vi "Encode Remaining Length.vi"(11 "Remaining Length (bytes)":u32) -> (2 "Valid length":bool, 3 "Encoded Remaining Length":u8[](array[numeric]) format="%02x")   [LabVIEW 2013, in "ControlPacket.lvclass"]
uses:
  ControlPacket.lvclass
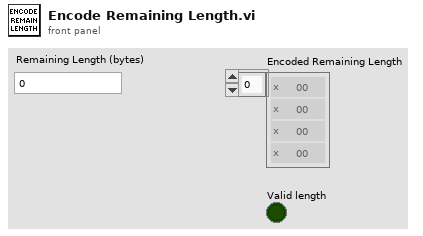
[diagram p1: front panel]
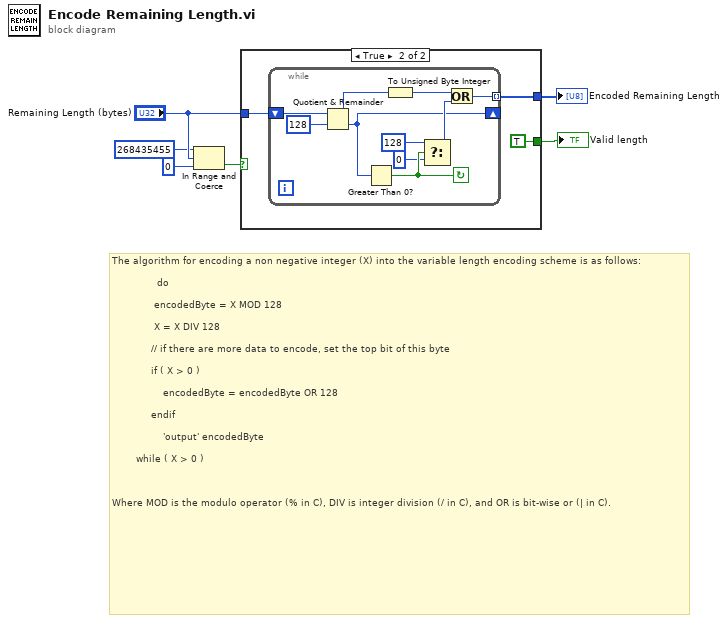
[diagram p0: block diagram]
diagram:
  # "The algorithm for encoding a non negative integer (X) into the variable length encoding scheme is as follows:\n\n               do\n\n              encodedByte = X MOD 128\n\n              X = X DIV 128\n\n             // if there are more data to encode, set the top bit of this byte\n\n             if ( X > 0 )\n\n                 encodedByte = encodedByte OR 128\n\n             endif\n\n                 'output' encodedByte\n\n        while ( X > 0 )\n\n \n\nWhere MOD is the modulo operator (% in C), DIV is integer division (/ in C), and OR is bit-wise or (| in C)."
  n1 = In Range and Coerce(upper limit=u32 268435455, x="Remaining Length (bytes)", lower limit=u32 0) -> (In Range?=w2:bool)  [unwired: 1 out]
  n2 = case shown="True" w2 {
    tunnel: [_ w9] -> w6
    tunnel: "Remaining Length (bytes)" -> [_ w8]
    tunnel: [_ TRUE] -> w1
    frame False {
    }
    frame True {
      n3 = while {
        shift-right: [w10] -> _
        shift-left: w8 -> [w19]
        tunnel: [w15] -> w9 mode=indexing
        stop <- w14 continue-if-true
        n4 = Quotient & Remainder(x=w19, y=u32 128) -> (x-y*floor(x/y)=w18:u32, floor(x/y)=w10:u32)
        n5 = Greater Than 0?(x=w10) -> (x > 0?=w14:bool)
        n6 = To Unsigned Byte Integer(number=w18) -> (unsigned 8bit integer=w16:u8)
        n7 = Select(t=u8 128 ("y"), s=w14, f=u8 0) -> (s? t:f=w11:u8)
        n8 = Or(x=w16, y=w11) -> (x .or. y?=w15:u8)
      }
    }
  }
  "Encoded Remaining Length" <- w6
  "Valid length" <- w1
